vi "Test Measurement Class.vi"() -> ()   [LabVIEW 2013]
doc: "This VI tests the functionality of the measurement class, specifically whether it successfully connects to the database file, writes data to the file, and shuts down properly."
uses:
  Classes/DbMeasurement/DbMeasurement.lvclass
  Classes/DbMeasurement/DbMeasurement.lvclass/DbMeasurement.ctl
panel:
  in  "Mood":string="Good"
  in  "Name":string="Nathan"
  in  "Stop Button":bool
  in  "Record":bool
  in  "connection information":path=path "C:/Users/Nathan/Documents/LV_testRig-Dev/Data/measurement_data.udl"
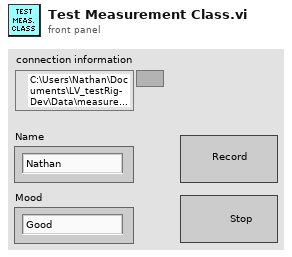
[diagram p1: front panel]
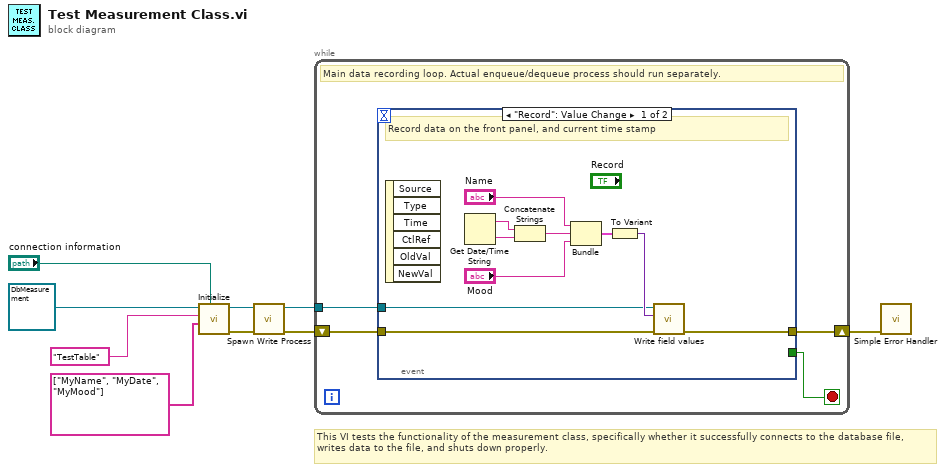
[diagram p0: block diagram]
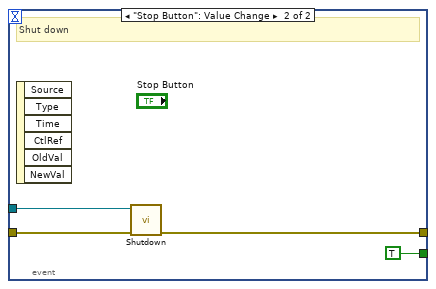
[diagram p2: hidden frame]
diagram:
  # "This VI tests the functionality of the measurement class, specifically whether it successfully connects to the database file, writes data to the file, and shuts down properly."
  n1 = call "Initialize.vi"("connection information"="connection information", "columns"=string[] ["MyName", "MyDate", "MyMood"], "table"="TestTable", "DbMeasurement in"=refnum<class "DbMeasurement.lvclass"> refnum ("DbMeasurement.lvclass")) -> ("error out"=w4:errorcluster, "DbMeasurement out"=w3:refnum<class "DbMeasurement.lvclass">)  [unwired: 6 in]
  n2 = call "Spawn Write Process.vi"("error in (no error)"=w4, "DbMeasurement in"=w3) -> ("error out"=w5:errorcluster, "DbMeasurement out"=w6:refnum<class "DbMeasurement.lvclass">)  [unwired: 8 in]
  n3 = while {
    shift-right: [w12] -> w7
    shift-left: w5 -> [w13]
    tunnel: w6 -> [w11]
    stop <- w10 stop-if-true
    # "Main data recording loop. Actual enqueue/dequeue process should run separately."
    n4 = event shown="[0] \"Record\": Value Change" {
      selector: _ -> [_ _]
      dyn-events: _ -> [_ _]
      timeout: _ -> [_ _]
      tunnel: w13 -> [w18 w27]
      tunnel: [w19 w25] -> w12
      tunnel: w11 -> [w17 w26]
      tunnel: [_ TRUE] -> w10
      event "Record": Value Change {
        # "Record data on the front panel, and current time stamp"
        n5 = event-data() -> ()  [unwired: 1 in, 6 out]
        n6 = Get Date/Time String() -> (date string=w16:string, time string=w15:string)  [unwired: 3 in]
        n7 = Concatenate Strings(w16, w15) -> (w14:string)
        n8 = Bundle("Name"="Name", w14, "Mood"="Mood") -> (w21:cluster{"Name":string, string, "Mood":string})  [unwired: 1 in]
        n9 = To Variant(anything=w21) -> (Variant=w20:variant)
        n10 = call "Write field values.vi"("error in (no error)"=w18, "field values"=w20, "DbMeasurement in"=w17) -> ("error out"=w19:errorcluster)  [unwired: 7 in, 1 out]
      }
      event "Stop Button": Value Change {
        # "Shut down"
        n11 = event-data() -> ()  [unwired: 1 in, 6 out]
        n12 = call "Shutdown.vi"("error in (no error)"=w27, "DbMeasurement in"=w26) -> ("error out"=w25:errorcluster)  [unwired: 8 in, 1 out]
      }
    }
  }
  n13 = call <vilib>:"Simple Error Handler.vi"("error in (no error)"=w7) -> ()  [unwired: 4 in, 5 out]
